vi "Result.Create Summary Result form 1D Results.vi"(10 "Abort":bool, 11 "Results":T2[](array[typedef]) {"Status" items=["LOG", "PASS", "FAIL", "ERROR"]}) -> (0 "Desc":string, 1 "Result":string, 2 "Code":i32, 3 "Color":u32(colorbox)=13816530, 4 "Fault Result":T2 {"Status" items=["LOG", "PASS", "FAIL", "ERROR"]}, 5 "Result.Result":T1=enum."Completed")   [LabVIEW 2019]
uses:
  Result.Measurement Item.ctl
  Result.Measurement and Attribute Item Status.ctl
  Result XML/TestResult.Symptom.State.ctl
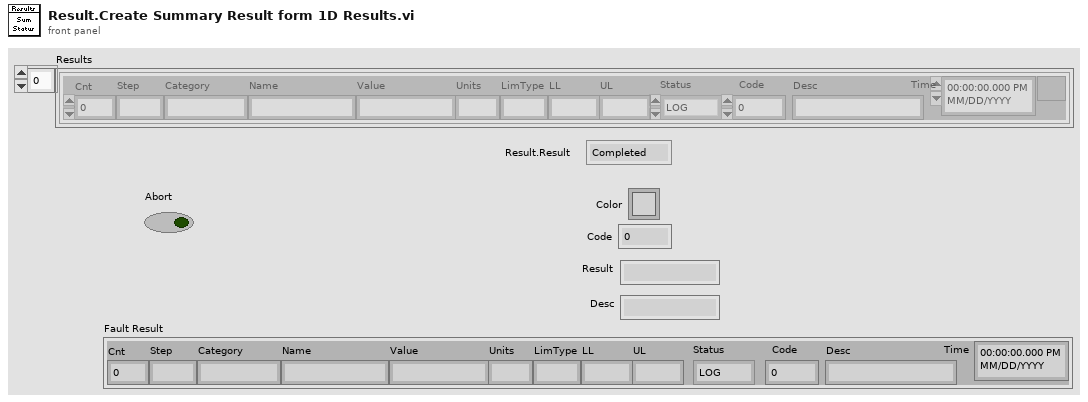
[diagram p1: front panel]
types:
  T1 = typedef "TestResult.Symptom.State.ctl" = enum16{"Pass", "Fail", "Error", "Aborted", "Completed", "Logged"}
  T2 = typedef "Result.Measurement Item.ctl" = cluster{"Cnt":i32, "Step":string, "Category":string, "Name":string, "Value":string, "Units":string, "LimType":string, "LL":string, "UL":string, "Status":T3, "Code":i32, "Desc":string, "Time":timestamp}
  T3 = typedef "Result.Measurement and Attribute Item Status.ctl" = i32
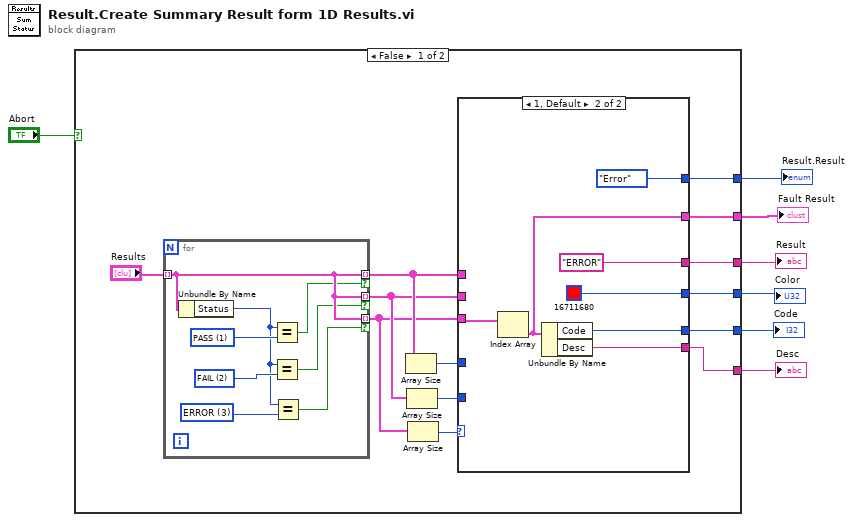
[diagram p0: block diagram]
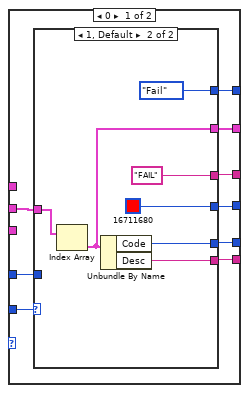
[diagram p2: hidden frame]
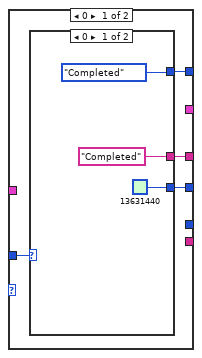
[diagram p3: hidden frame]
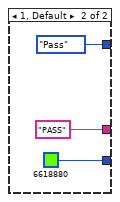
[diagram p4: hidden frame]
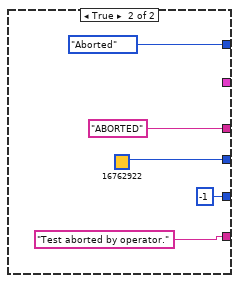
[diagram p5: hidden frame]
diagram:
  n1 = case shown="False" "Abort" {
    tunnel: [w15 "ABORTED" ("y")] -> w7
    tunnel: [w12 -1 ("Code")] -> w6
    tunnel: [w11 "Test aborted by operator." ("y")] -> w5
    tunnel: [w10 u32 16762922] -> w4
    tunnel: [w9 _] -> w3
    tunnel: [w8 TestResult.Symptom.State."Aborted" ("Result.Result")] -> w2
    frame False {
      n2 = for {
        tunnel: "Results" -> [w57] mode=indexing
        tunnel: [w57] -> w18 mode=indexing if=w56
        tunnel: [w57] -> w17 mode=indexing if=w55
        tunnel: [w57] -> w16 mode=indexing if=w54
        w60 = T3 3 items=["LOG", "PASS", "FAIL", "ERROR"] ("y")
        w59 = T3 2 items=["LOG", "PASS", "FAIL", "ERROR"] ("y")
        w61 = T3 1 items=["LOG", "PASS", "FAIL", "ERROR"] ("y")
        n3 = Unbundle By Name(w57) -> ("Status"=w58:T3)
        n4 = Equal?(x=w58, y=w61) -> (x = y?=w56:bool)
        n5 = Equal?(x=w58, y=w59) -> (x = y?=w55:bool)
        n6 = Equal?(x=w58, y=w60) -> (x = y?=w54:bool)
      }
      n7 = Array Size(array=w18) -> (size(s)=w14:i32)
      n8 = Array Size(array=w17) -> (size(s)=w13:i32)
      n9 = Array Size(array=w16) -> (size(s)=w19:i32)
      n10 = case shown="1, Default" w19 {
        tunnel: w18 -> [_ _]
        tunnel: w17 -> [w28 _]
        tunnel: w16 -> [_ w52]
        tunnel: [w26 "ERROR" ("y")] -> w15
        tunnel: w14 -> [w23 _]
        tunnel: w13 -> [w29 _]
        tunnel: [w25 w51] -> w12
        tunnel: [w24 w50] -> w11
        tunnel: [w27 u32 16711680] -> w10
        tunnel: [w22 w48] -> w9
        tunnel: [w21 TestResult.Symptom.State."Error" ("Result.Result")] -> w8
        frame 0 {
          n11 = case shown="1, Default" w29 {
            tunnel: [w31 "FAIL" ("y")] -> w26
            tunnel: w28 -> [_ w42]
            tunnel: [_ w45] -> w25
            tunnel: [_ w44] -> w24
            tunnel: [w32 u32 16711680] -> w27
            tunnel: w23 -> [w33 _]
            tunnel: [_ w41] -> w22
            tunnel: [w30 TestResult.Symptom.State."Fail" ("Result.Result")] -> w21
            frame 0 {
              n12 = case shown="0" w33 {
                tunnel: [u32 13631440 u32 6618880] -> w32
                tunnel: ["Completed" ("y") "PASS" ("y")] -> w31
                tunnel: [TestResult.Symptom.State."Completed" ("Result.Result") TestResult.Symptom.State."Pass" ("Result.Result")] -> w30
                frame 0 {
                }
                frame 1, Default {
                }
              }
            }
            frame 1, Default {
              n13 = Index Array(array=w42) -> (element=w41:T2)  [unwired: 1 in]
              n14 = Unbundle By Name(w41) -> ("Code"=w45:i32, "Desc"=w44:string)
            }
          }
        }
        frame 1, Default {
          n15 = Index Array(array=w52) -> (element=w48:T2)  [unwired: 1 in]
          n16 = Unbundle By Name(w48) -> ("Code"=w51:i32, "Desc"=w50:string)
        }
      }
    }
    frame True {
    }
  }
  "Color" <- w4
  "Code" <- w6
  "Result" <- w7
  "Desc" <- w5
  "Fault Result" <- w3
  "Result.Result" <- w2
